vi "serialization test.vi"() -> ()   [LabVIEW 2013, in "execution interface tests.lvlib"]
uses:
  execution interface tests.lvlib
  Engine Configuration/Tag Info.ctl
  <vilib>/NI/Tag Bus/tag/tag descriptor.lvclass
  Engine Configuration/engine configuration.lvclass
  <vilib>/NI/Tag Bus Module Framework/channel/TBM channel.lvclass
  <vilib>/NI/Configuration Framework/serializable configuration/NISE_CEF_serializable configuration.lvclass
panel:
  out "data":string
  out "raw tag data":T1[](array[typedef])
  out "error out":errorcluster
  out "ok?":bool
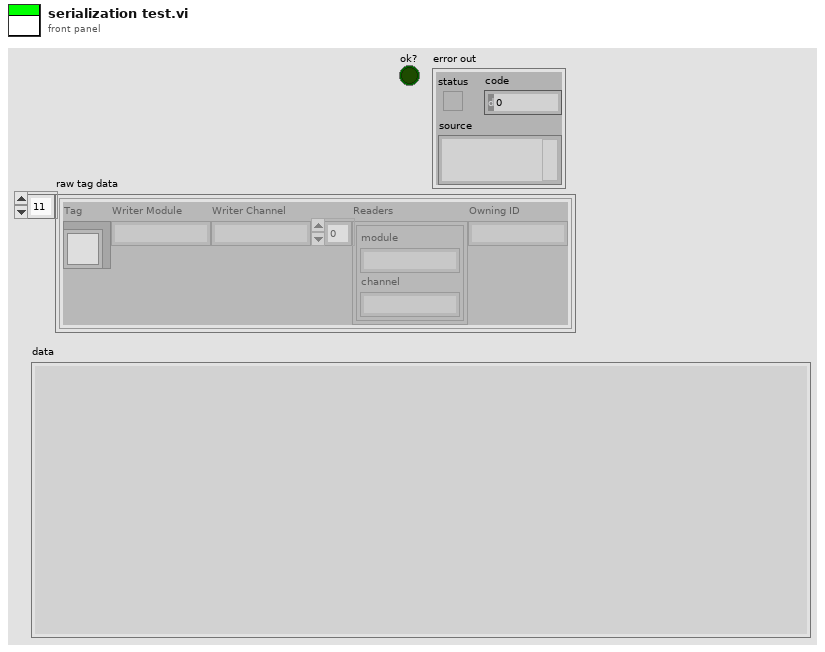
[diagram p1: front panel]
types:
  T1 = typedef "engine configuration.lvclass/Tag Info.ctl" = cluster{"Tag":refnum<class "tag descriptor.lvclass">, "Writer Module":string, "Writer Channel":string, "Readers":cluster{"module":string, "channel":string}[], "Owning ID":string}
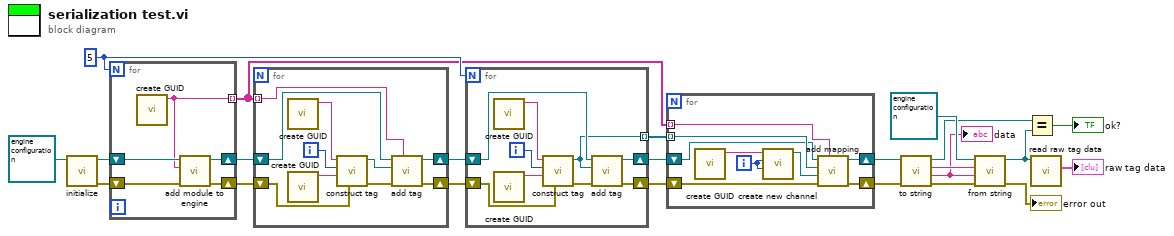
[diagram p0: block diagram]
diagram:
  w9 = 5
  n1 = call <vilib>:"initialize.vi"("configuration in"=refnum<class "engine configuration.lvclass"> refnum ("engine configuration")) -> ("error out"=w14:errorcluster, "configuration out"=w15:refnum<class "engine configuration.lvclass">)  [unwired: 8 in, 1 out]
  n2 = for {
    N: w9 -> [_]
    shift-right: [w26] -> w13
    shift-left: w15 -> [w28]
    shift-right: [w25] -> w12
    shift-left: w14 -> [w27]
    tunnel: [w24] -> w7 mode=indexing
    n3 = call <vilib>:"create GUID.vi"() -> ("uuid"=w24:string)  [unwired: 10 in, 1 out]
    n4 = call-dynamic "add module to engine.vi"("error in"=w27, "module ID"=w24, "engine configuration in"=w28) -> ("error out"=w25:errorcluster, "engine configuration out"=w26:refnum<class "engine configuration.lvclass">)  [unwired: 7 in]
  }
  n5 = for {
    tunnel: w7 -> [w38] mode=indexing
    shift-right: [w36] -> w11
    shift-left: w13 -> [w35]
    shift-right: [w37] -> w10
    shift-left: w12 -> [w34]
    i -> [w31]
    n6 = call <vilib>:"create GUID.vi"() -> ("uuid"=w29:string)  [unwired: 10 in, 1 out]
    n7 = call <vilib>:"create GUID.vi"() -> ("uuid"=w30:string)  [unwired: 10 in, 1 out]
    n8 = call <vilib>:"construct tag.vi"("error in"=w34, "metadata"=w30, "data type"=w31, "name"=w29) -> ("error out"=w33:errorcluster, "system tag out"=w32:refnum<class "tag descriptor.lvclass">)  [unwired: 6 in]
    n9 = call "add tag.vi"("owner ID"=w38, "error in"=w33, "tag descriptor"=w32, "engine configuration in"=w35) -> ("error out"=w37:errorcluster, "engine configuration out"=w36:refnum<class "engine configuration.lvclass">)  [unwired: 6 in]
  }
  n10 = for {
    N: w9 -> [_]
    shift-right: [w46] -> w6
    shift-left: w11 -> [w45]
    shift-right: [w47] -> w4
    shift-left: w10 -> [w44]
    tunnel: [w41] -> w8 mode=indexing
    i -> [w42]
    n11 = call <vilib>:"create GUID.vi"() -> ("uuid"=w40:string)  [unwired: 10 in, 1 out]
    n12 = call <vilib>:"create GUID.vi"() -> ("uuid"=w39:string)  [unwired: 10 in, 1 out]
    n13 = call <vilib>:"construct tag.vi"("error in"=w44, "metadata"=w39, "data type"=w42, "name"=w40) -> ("error out"=w43:errorcluster, "system tag out"=w41:refnum<class "tag descriptor.lvclass">)  [unwired: 6 in]
    n14 = call "add tag.vi"("error in"=w43, "tag descriptor"=w41, "engine configuration in"=w45) -> ("error out"=w47:errorcluster, "engine configuration out"=w46:refnum<class "engine configuration.lvclass">)  [unwired: 7 in]
  }
  n15 = for {
    tunnel: w8 -> [w56] mode=indexing
    tunnel: w7 -> [w55] mode=indexing
    shift-right: [w53] -> w3
    shift-left: w6 -> [w54]
    shift-right: [w52] -> w5
    shift-left: w4 -> [w51]
    i -> [w49]
    n16 = call <vilib>:"create GUID.vi"() -> ("uuid"=w48:string)  [unwired: 10 in, 1 out]
    n17 = call <vilib>:"create new channel.vi"("channel classification"=w49, "data type"=w49, "channel name"=w48) -> ("channel"=w50:refnum<class "TBM channel.lvclass">)  [unwired: 8 in]
    n18 = call "add mapping.vi"("owner ID"=w55, "error in"=w51, "channel"=w50, "tag descriptor"=w56, "engine configuration"=w54) -> ("error out"=w52:errorcluster, "engine configuration out"=w53:refnum<class "engine configuration.lvclass">)  [unwired: 5 in]
  }
  n19 = call-dynamic "to string.vi"("error in"=w5, "engine configuration in"=w3) -> ("error out"=w21:errorcluster, "data"=w19:string, "version"=w20:string, "engine configuration out"=w18:refnum<class "engine configuration.lvclass">)  [unwired: 6 in]
  "data" <- w19
  n20 = call-dynamic "from string.vi"("error in"=w21, "data"=w19, "version"=w20, "engine configuration in"=refnum<class "engine configuration.lvclass"> refnum ("engine configuration")) -> ("error out"=→"error out":errorcluster, "engine configuration out"=w2:refnum<class "engine configuration.lvclass">)  [unwired: 6 in]
  n21 = Equal?(x=w18, y=w2) -> (x = y?=→"ok?":bool)
  n22 = call "read raw tag data.vi"("engine configuration in"=w2) -> ("raw tag data"=→"raw tag data":T1[])  [unwired: 8 in, 2 out]
